vi "set pipelining.vi"(8 "error in (no error)":errorcluster, 10 "enabled?":bool, 11 "Redis Pipelining TCP Client in":refnum<class "Redis Pipelining TCP Client.lvclass">) -> (0 "error out":errorcluster, 3 "Redis Pipelining TCP Client out":refnum<class "Redis Pipelining TCP Client.lvclass">)   [LabVIEW 2019, in "Redis Client for LabVIEW.lvlib" / "Redis Pipelining TCP Client.lvclass"]
uses:
  Redis Pipelining TCP Client.lvclass
  Redis Pipelining TCP Client.lvclass/Redis Pipelining TCP Client.ctl
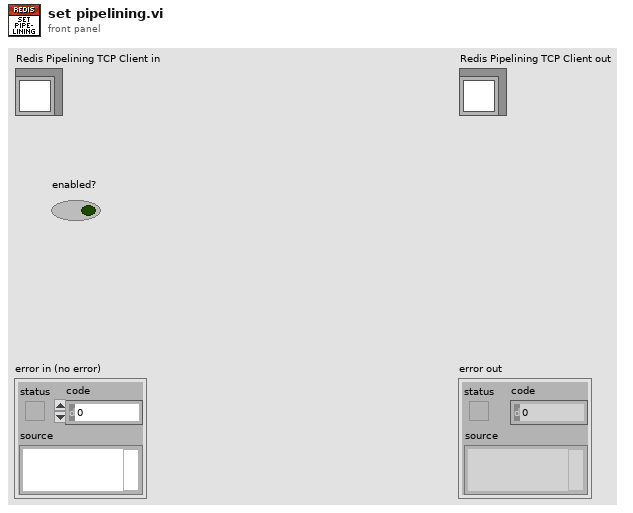
[diagram p1: front panel]
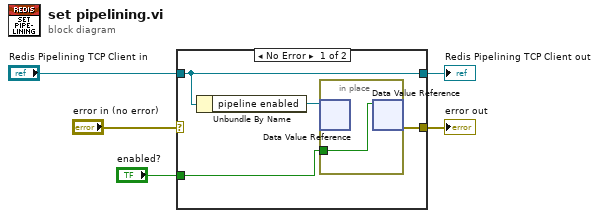
[diagram p0: block diagram]
diagram:
  n1 = case shown="No Error" "error in (no error)" {
    selector: "error in (no error)" -> [_ w12]
    tunnel: [w6 w12] -> w4
    tunnel: [w9 w11] -> w2
    tunnel: "Redis Pipelining TCP Client in" -> [w9 w11]
    tunnel: "enabled?" -> [w7 _]
    frame No Error {
      n2 = Unbundle By Name(w9) -> ("pipeline enabled"=w8:refnum<data-value>)
      n3 = in-place {
        in-place-border: w7 -> [w10]
        n4 = in-place-dvr #1(w8) -> ()  [unwired: 2 out]
        n5 = in-place-dvr #1(w10) -> (w6:errorcluster)  [unwired: 1 out]
      }
    }
    frame Error {
    }
  }
  "error out" <- w4
  "Redis Pipelining TCP Client out" <- w2
